vi "JUnit Basic.vi"() -> ()   [LabVIEW 2013]
doc: "This example illustrates the basic usage of <B>JUnit XML</B>."
uses:
  JUnit XML/Test Suite/Test Suite.lvclass
  <vilib>/xml/Close Reference(Node).vi
  <vilib>/xml/NI_XML.lvlib
  JUnit XML/Test Case/Test Case.lvclass
  <resource>/objmgr/DOMUserDefRef.rc
panel:
  out "XML":string
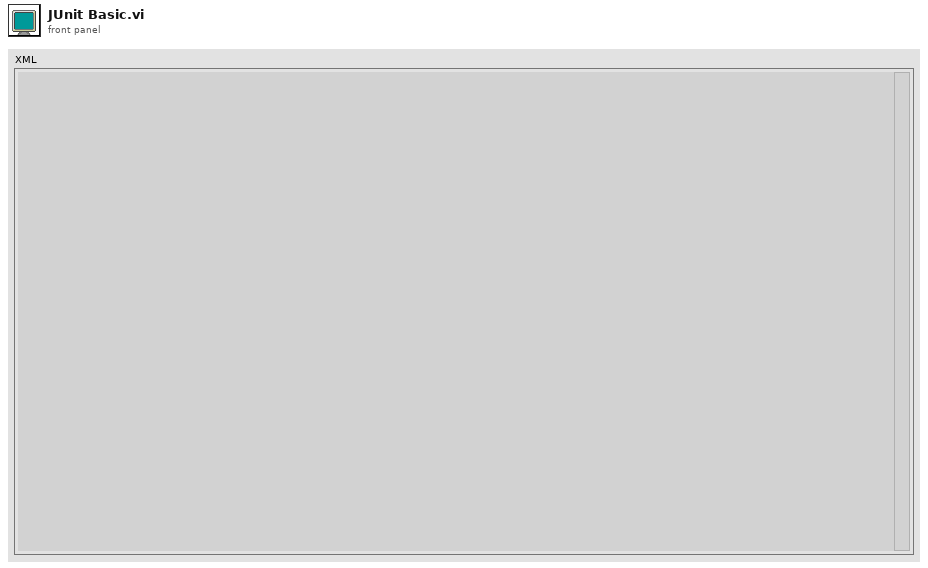
[diagram p1: front panel]
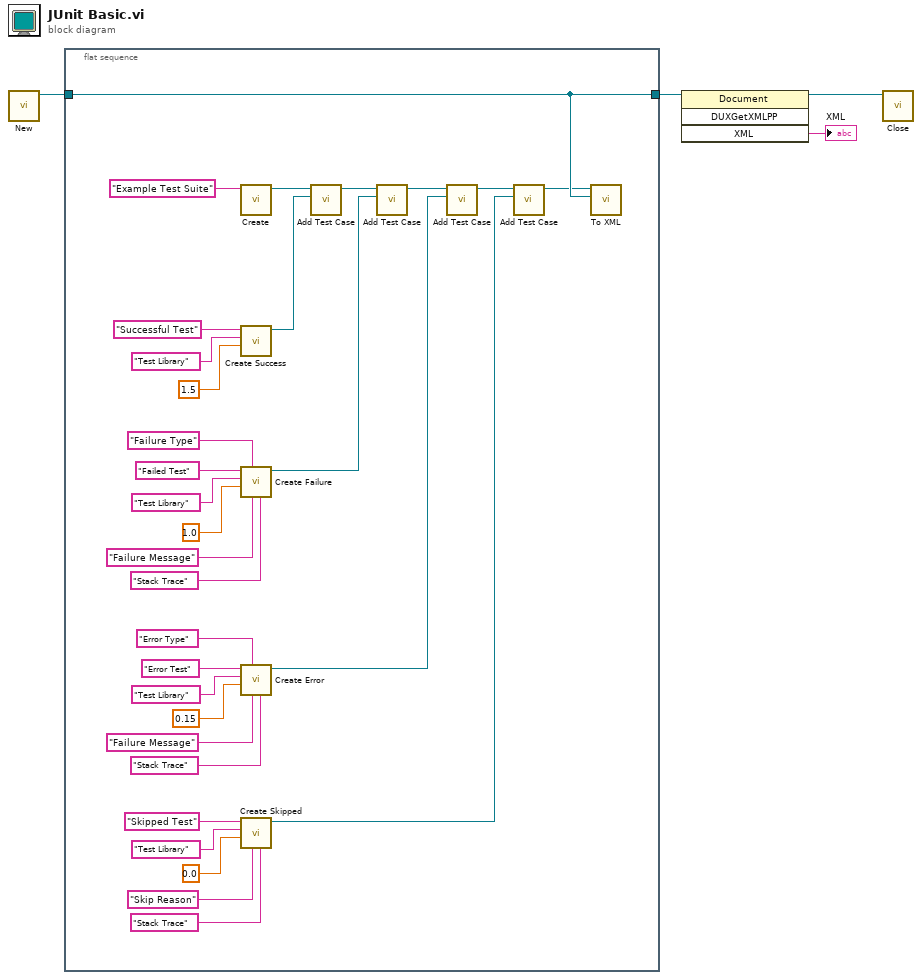
[diagram p0: block diagram]
diagram:
  n1 = call <vilib>:"New.vi"() -> ("DOM document out"=w4:refnum<k20>)  [unwired: 8 in, 1 out]
  n2 = flat-sequence {
    tunnel: w4 -> [w29]
    tunnel: [w29] -> w2
    frame #0 {
      n3 = call "Create.vi"("Name"="Example Test Suite") -> ("Test Suite"=w31:refnum<class "Test Suite.lvclass">)  [unwired: 9 in, 1 out]
      n4 = call "Create Success.vi"("Time"=1.5, "Classname"="Test Library", "Name"="Successful Test") -> ("Test Case"=w30:refnum<class "Test Case.lvclass">)  [unwired: 7 in, 1 out]
      n5 = call "Create Failure.vi"("Stack Trace"="Stack Trace", "Message"="Failure Message", "Type"="Failure Type", "Time"=1.0, "Classname"="Test Library", "Name"="Failed Test") -> ("Test Case"=w21:refnum<class "Test Case.lvclass">)  [unwired: 4 in, 1 out]
      n6 = call "Create Error.vi"("Stack Trace"="Stack Trace", "Message"="Failure Message", "Type"="Error Type", "Time"=0.15, "Classname"="Test Library", "Name"="Error Test") -> ("Test Case"=w13:refnum<class "Test Case.lvclass">)  [unwired: 4 in, 1 out]
      n7 = call "Create Skipped.vi"("Stack Trace"="Stack Trace", "Message"="Skip Reason", "Time"=0.0, "Classname"="Test Library", "Name"="Skipped Test") -> ("Test Case"=w5:refnum<class "Test Case.lvclass">)  [unwired: 5 in, 1 out]
      n8 = call "Add Test Case.vi"("Test Case"=w30, "Test Suite in"=w31) -> ("Test Suite out"=w22:refnum<class "Test Suite.lvclass">)  [unwired: 8 in, 1 out]
      n9 = call "Add Test Case.vi"("Test Case"=w21, "Test Suite in"=w22) -> ("Test Suite out"=w14:refnum<class "Test Suite.lvclass">)  [unwired: 8 in, 1 out]
      n10 = call "Add Test Case.vi"("Test Case"=w13, "Test Suite in"=w14) -> ("Test Suite out"=w7:refnum<class "Test Suite.lvclass">)  [unwired: 8 in, 1 out]
      n11 = call "Add Test Case.vi"("Test Case"=w5, "Test Suite in"=w7) -> ("Test Suite out"=w6:refnum<class "Test Suite.lvclass">)  [unwired: 8 in, 1 out]
      n12 = call-dynamic "To XML.vi"("Parent"=w29, "Test Suite in"=w6) -> ()  [unwired: 9 in, 1 out]
    }
  }
  n13 = invoke class="Document" method="DUXGetXMLPP"(reference=w2) -> (reference out=w3:refnum<k20>, "XML"=→"XML":string)  [unwired: 3 in, 2 out]
  n14 = call-poly <vilib>:"Close.vi"("node"=w3) -> ()  [unwired: 8 in, 1 out]
